vi "Check Move.vi"(5 "source vi name":string, 6 "count power of 2":i16, 7 "buffer count":u64 format="%d elements", 8 "error in (no error)":errorcluster, 9 "offset (0)":u64 format="%d bytes", 10 "move count (-1: rest)":i64=-1 format="%d elements", 11 "Pointer in":refnum<class "Pointer.lvclass">) -> (0 "error out":errorcluster, 1 "offset":u64 format="%d bytes", 2 "count":u64 format="%d elements", 3 "Pointer out":refnum<class "Pointer.lvclass">)   [LabVIEW 2016, in "Memory Manager.lvlib" / "Pointer.lvclass"]
uses:
  Pointer.lvclass
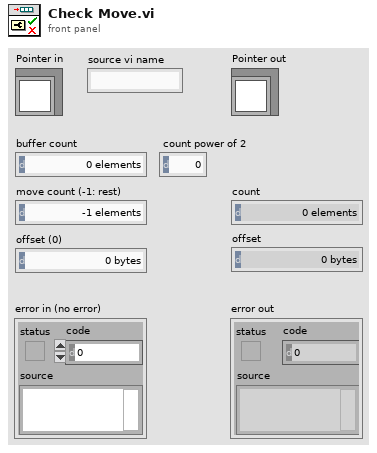
[diagram p1: front panel]
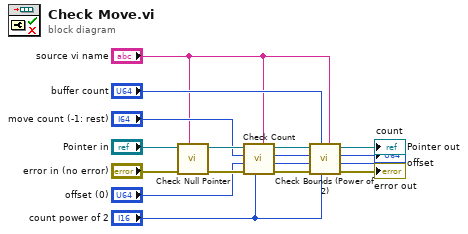
[diagram p0: block diagram]
diagram:
  n1 = call "Check Null Pointer.vi"("source vi name"="source vi name", "error in (no error)"="error in (no error)", "Pointer in"="Pointer in") -> ("error out"=w14:errorcluster, "Pointer out"=w15:refnum<class "Pointer.lvclass">)  [unwired: 7 in]
  n2 = call "Check Count.vi"("source vi name"="source vi name", "count power of 2"="count power of 2", "error in (no error)"=w14, "offset (0)"="offset (0)", "count (-1: rest)"="move count (-1: rest)", "Pointer in"=w15) -> ("error out"=w10:errorcluster, "offset"=w8:u64, "count"=w9:u64, "Pointer out"=w11:refnum<class "Pointer.lvclass">)  [unwired: 2 in]
  n3 = call "Check Bounds (Power of 2).vi"("source vi name"="source vi name", "count power of 2"="count power of 2", "buffer count"="buffer count", "error in (no error)"=w10, "offset (0)"=w8, "move count"=w9, "Pointer in"=w11) -> ("error out"=→"error out":errorcluster, "offset"=→"offset":u64, "move count"=→"count":u64, "Pointer out"=→"Pointer out":refnum<class "Pointer.lvclass">)  [unwired: 1 in]
